vi "MH_GetLibraryVersion.vi"(8 "error in (no error)":errorcluster) -> (0 "error out":errorcluster, 2 "Version":string, 3 "return type":i32)   [LabVIEW 2019]
uses:
  MH_DllPath_global.vi
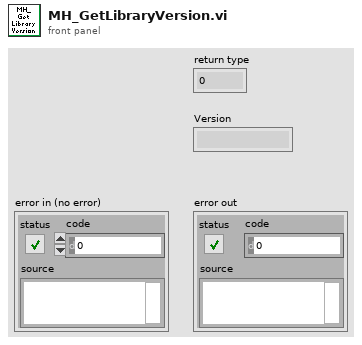
[diagram p1: front panel]
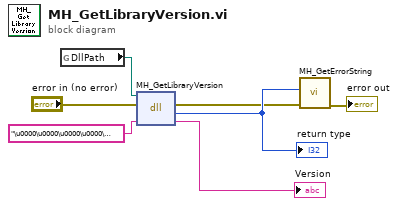
[diagram p0: block diagram]
diagram:
  n1 = global read "MH_DllPath_global.vi" "DllPath"() -> (w7:path)
  n2 = dll-call lib="MHLib64.dll" fn="MH_GetLibraryVersion"(path in=w7, error in="error in (no error)", "Version"="\u0000\u0000\u0000\u0000\u0000\u0000\u0000\u0000") -> (error out=w2:errorcluster, "return type"=w3:i32, "Version"=→"Version":string)  [unwired: 1 in, 1 out]
  "return type" <- w3
  n3 = call "MH_GetErrorString.vi"("error in (no error)"=w2, "code"=w3) -> ("error out"=→"error out":errorcluster)  [unwired: 7 in, 2 out]
